vi "AIselector.vi"(8 "I/O element":T1(ring)) -> (3 "value":i16)   [LabVIEW 2024]
uses:
  <vilib>/eio/EIONode/EIONode.xnode
  <vilib>/rvi/eio/common/nirviEmuTemplateMethod_errors.vi
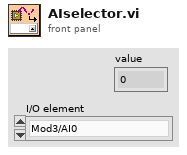
[diagram p1: front panel]
types:
  T1 = enum16{"Mod3/AI0", "Mod3/AI1", "Mod3/AI2", "Mod3/AI3", "Mod3/AI4", "Mod3/AI5", "Mod3/AI6", "Mod3/AI7"}
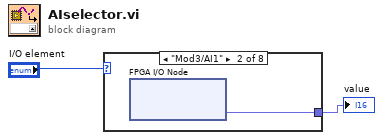
[diagram p0: block diagram]
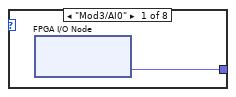
[diagram p2: hidden frame]
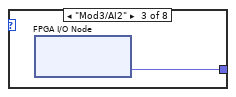
[diagram p3: hidden frame]
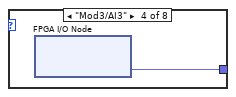
[diagram p4: hidden frame]
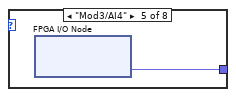
[diagram p5: hidden frame]
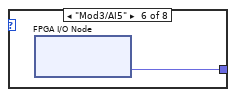
[diagram p6: hidden frame]
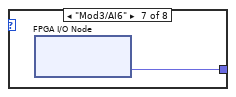
[diagram p7: hidden frame]
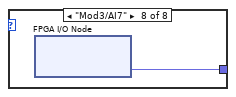
[diagram p8: hidden frame]
diagram:
  n1 = case shown="\"Mod3/AI1\"" "I/O element" {
    tunnel: [w3 w4 w5 w6 w7 w8 w9 w10] -> w1
    frame "Mod3/AI0" {
      n2 = xnode "FPGA I/O Node"() -> ("Mod3/AI0"=w3:fxp<+/-,21,-4>)  [unwired: 2 in, 2 out]
    }
    frame "Mod3/AI1" {
      n3 = xnode "FPGA I/O Node"() -> ("Mod3/AI1"=w4:fxp<+/-,21,-4>)  [unwired: 2 in, 2 out]
    }
    frame "Mod3/AI2" {
      n4 = xnode "FPGA I/O Node"() -> ("Mod3/AI2"=w5:fxp<+/-,21,-4>)  [unwired: 2 in, 2 out]
    }
    frame "Mod3/AI3" {
      n5 = xnode "FPGA I/O Node"() -> ("Mod3/AI3"=w6:fxp<+/-,21,-4>)  [unwired: 2 in, 2 out]
    }
    frame "Mod3/AI4" {
      n6 = xnode "FPGA I/O Node"() -> ("Mod3/AI4"=w7:fxp<+/-,21,-4>)  [unwired: 2 in, 2 out]
    }
    frame "Mod3/AI5" {
      n7 = xnode "FPGA I/O Node"() -> ("Mod3/AI5"=w8:fxp<+/-,21,-4>)  [unwired: 2 in, 2 out]
    }
    frame "Mod3/AI6" {
      n8 = xnode "FPGA I/O Node"() -> ("Mod3/AI6"=w9:fxp<+/-,21,-4>)  [unwired: 2 in, 2 out]
    }
    frame "Mod3/AI7" {
      n9 = xnode "FPGA I/O Node"() -> ("Mod3/AI7"=w10:fxp<+/-,21,-4>)  [unwired: 2 in, 2 out]
    }
  }
  "value" <- w1
